vi "ShiftArrElBoolGen.vi"(8 "ErrorIn(No Error)":errorcluster caption="entrée d'erreur (pas d'erreur)", 9 "Index":i32, 10 "Dir(DownFalse)":bool, 11 "Array In":bool[](array[boolean])) -> (0 "sortie d'erreur":errorcluster, 1 "NewIndex":i32, 3 "Array Out":bool[](array[boolean]))   [LabVIEW 2019]
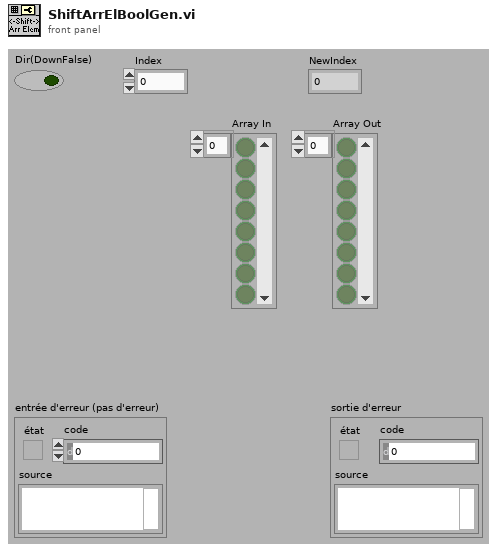
[diagram p1: front panel]
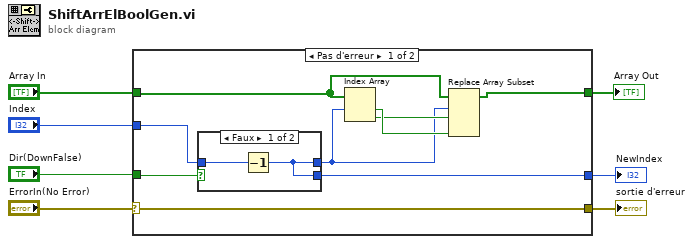
[diagram p0: block diagram]
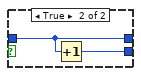
[diagram p2: hidden frame]
diagram:
  n1 = case shown="Pas d'erreur" "ErrorIn(No Error)" {
    selector: "ErrorIn(No Error)" -> [w16 w23]
    tunnel: [w16 w23] -> w6
    tunnel: "Array In" -> [w10 w22]
    tunnel: [w9 w22] -> w4
    tunnel: "Dir(DownFalse)" -> [w12 _]
    tunnel: "Index" -> [w11 w21]
    tunnel: [w8 w21] -> w1
    frame No Error {
      n2 = case shown="Faux" w12 {
        tunnel: w11 -> [w18 w20]
        tunnel: [w17 w20] -> w13
        tunnel: [w17 w19] -> w8
        frame False {
          n3 = Decrement(x=w18) -> (x-1=w17:i32)
        }
        frame True {
          n4 = Increment(x=w20) -> (x+1=w19:i32)
        }
      }
      n5 = Index Array(array=w10, index #1=w13) -> (element #1=w15:bool, element #2=w14:bool)  [unwired: 1 in]
      n6 = Replace Array Subset(array=w10, new element #1=w14, index #1=w13, new element #2=w15) -> (w9:bool[])  [unwired: 1 in]
    }
    frame Error {
    }
  }
  "sortie d'erreur" <- w6
  "Array Out" <- w4
  "NewIndex" <- w1
